vi "Numeric Functions Mersenne Prime.vi"() -> ()   [LabVIEW 2019]
panel:
  out "Mersenne Prime":dbl
  in  "Prime Number n":dbl
  # "Challenge:\nMersenne prime. Write a program that accepts a prime number n and uses it to calculate a Mersenne prime, which has the form 2^n - 1"
  # "Try it: Enter a prime number in the \"Prime Number n\" box and hit Run."
  # "You will probably need:\nControls, indicators, and constants, numeric functions."
  # "Open the block diagram to see a possible solution."
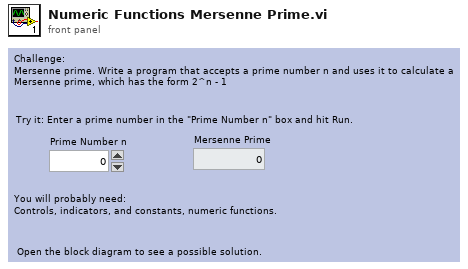
[diagram p1: front panel]
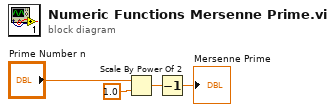
[diagram p0: block diagram]
diagram:
  n1 = Scale By Power Of 2(n="Prime Number n", x=1.0) -> (x*2^n=w2:dbl)
  n2 = Decrement(x=w2) -> (x-1=→"Mersenne Prime":dbl)
